vi "New.vi"(8 "Error In":errorcluster, 11 "Content":string) -> (0 "Error Out":errorcluster, 3 "Text":refnum<class "Text.lvclass">)   [LabVIEW 2018, in "Toolkit.lvlib" / "Tokens.lvlib" / "Text.lvclass"]
uses:
  Text.lvclass
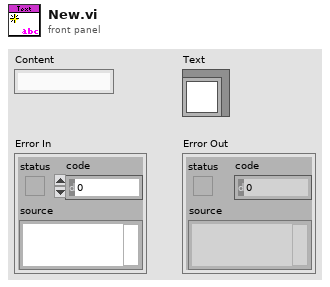
[diagram p1: front panel]
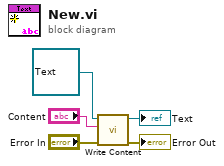
[diagram p0: block diagram]
diagram:
  n1 = call-dynamic "Write Content.vi"("Error In"="Error In", "Content"="Content", "Contentable In"=refnum<class "Text.lvclass"> refnum ("Mustache.lvlib:Tokens.lvlib:Text.lvclass")) -> ("Error Out"=→"Error Out":errorcluster, "Contentable Out"=→"Text":refnum<class "Text.lvclass">)  [unwired: 7 in]
